vi "Test - Draw Lines 1.vi"() -> ()   [LabVIEW 2022 SP3, in "Raster.lvlib"]
uses:
  Raster.lvlib
  Screen Dimensions.ctl
  Point 2D.ctl
  <vilib>/Utility/High Resolution Relative Seconds.vi
  Draw Line.vi/ce09c930-e75c-45b5-9de7-7d3097d91b09.vi
  Draw Line.vi/8aa8c736-0805-475e-bbf3-9937bbefdeb4.vi
  Utility/Convert Pixels To Picture.vi/d601d993-a776-4dc8-89c7-357d8398c88c.vi
  Utility/Convert Pixels To Picture.vi/7816d0d6-8e4d-41a2-85ac-ed82f1435763.vi
  <vilib>/picture/picture.llb/Draw Unflattened Pixmap.vi
  <vilib>/picture/picture.llb/Draw True-Color Pixmap.vi
  Utility/Utility.lvlib
panel:
  out "Time [s]":dbl format="%.3p"
  in  "Numer Of Lines":i32=100
  out "new picture":picture
  # "(0,0)"
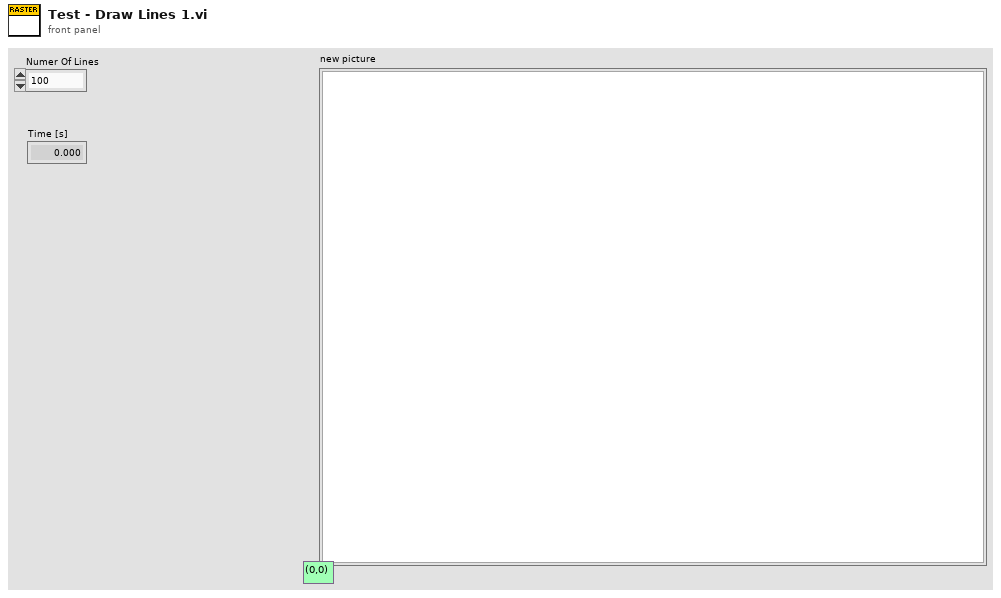
[diagram p1: front panel]
types:
  T1 = typedef "Raster.lvlib/Screen Dimensions.ctl" = cluster{"Width":u32, "Height":u32}
  T2 = typedef "Raster.lvlib/Point 2D.ctl" = cluster{"x":i32, "y":i32}
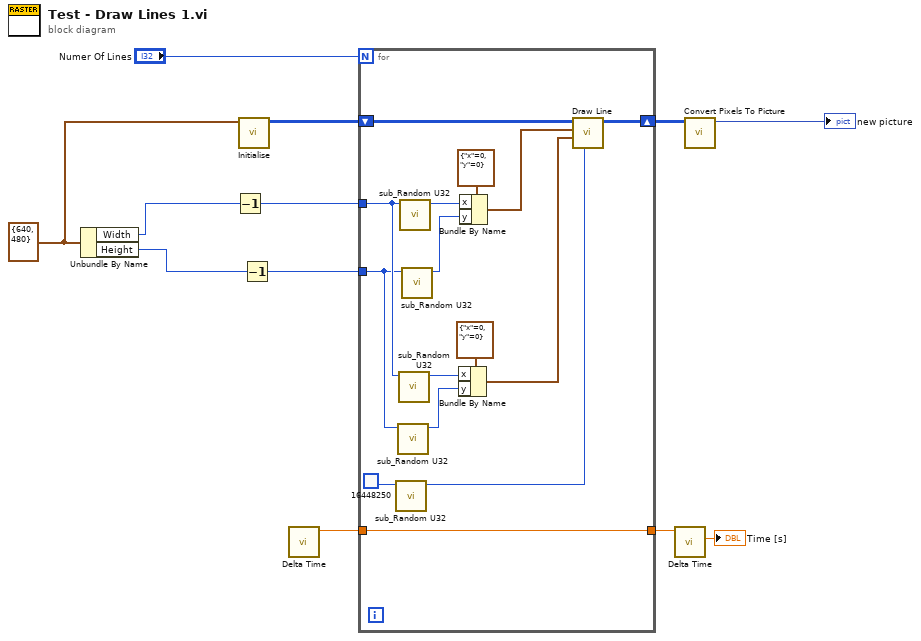
[diagram p0: block diagram]
diagram:
  w1 = T1 {"Width"=640, "Height"=480} ("Screen Dimensions")
  n1 = Unbundle By Name(w1) -> ("Width"=w3:u32, "Height"=w2:u32)
  n2 = Decrement(x=w3) -> (x-1=w8:u32)
  n3 = call "Initialise.vi"("Screen Dimensions"=w1) -> ("Pixel Data out"=w12:u32[][])  [unwired: 10 in]
  n4 = Decrement(x=w2) -> (x-1=w7:u32)
  n5 = call "Delta Time.vi"() -> ("Relative Seconds Out"=w6:dbl)  [unwired: 10 in, 1 out]
  n6 = for {
    N: "Numer Of Lines" -> [_]
    shift-right: [w26] -> w11
    shift-left: w12 -> [w27]
    tunnel: w8 -> [w18]
    tunnel: w7 -> [w17]
    tunnel: w6 -> [w15]
    tunnel: [w15] -> w5
    n7 = call <vilib>:"sub_Random U32.vi"("upper bound"=u32 16448250 ("Colour")) -> ("number"=w13:u32)  [unwired: 10 in]
    n8 = call <vilib>:"sub_Random U32.vi"("upper bound"=w17) -> ("number"=w21:u32)  [unwired: 10 in]
    n9 = call <vilib>:"sub_Random U32.vi"("upper bound"=w18) -> ("number"=w20:u32)  [unwired: 10 in]
    n10 = call <vilib>:"sub_Random U32.vi"("upper bound"=w18) -> ("number"=w23:u32)  [unwired: 10 in]
    n11 = call <vilib>:"sub_Random U32.vi"("upper bound"=w17) -> ("number"=w22:u32)  [unwired: 10 in]
    n12 = Bundle By Name(cluster=T2 {"x"=0, "y"=0} ("Point 1"), "x"=w20, "y"=w21) -> (w16:T2)
    n13 = Bundle By Name(cluster=T2 {"x"=0, "y"=0} ("Point 1"), "x"=w23, "y"=w22) -> (w24:T2)
    n14 = call "Draw Line.vi"("Colour"=w13, "Point 2"=w16, "Point 1"=w24, "Pixel Data in"=w27) -> ("Pixel Data out"=w26:u32[][])  [unwired: 7 in]
  }
  n15 = call "Delta Time.vi"("Relative Seconds In"=w5) -> ("Delta Time [s]"=→"Time [s]":dbl)  [unwired: 9 in, 1 out]
  n16 = call "Convert Pixels To Picture.vi"("Pixel Data in"=w11) -> ("2D Picture"=→"new picture":picture)  [unwired: 9 in, 1 out]
